vi "ROSmsg_createInd.vi"(9 "Names":string[](array[string]), 11 "SubVI Refnum":refnum<vi>) -> (1 "Exists?":bool, 2 "Control Refnums":refnum<vi>[](array[refnum]), 3 "SubVI Refnum 2":refnum<vi>)   [LabVIEW 2016]
doc: "Creates an indicator for a ROS message"
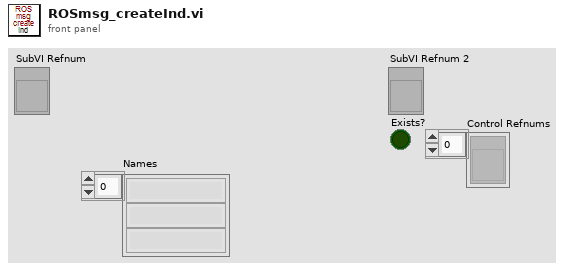
[diagram p1: front panel]
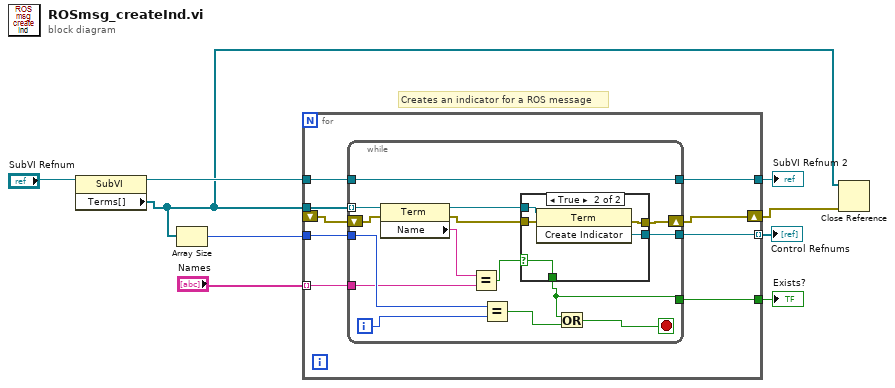
[diagram p0: block diagram]
diagram:
  # "Creates an indicator for a ROS message"
  n1 = property class="SubVI"(reference="SubVI Refnum") -> (reference out=w7:refnum<vi>, "Terms[]"=w1:refnum<vi>[])  [unwired: 1 in, 1 out]
  n2 = Array Size(array=w1) -> (size(s)=w8:i32)
  n3 = for {
    tunnel: w1 -> [w18]
    tunnel: w8 -> [w17]
    tunnel: w7 -> [w16]
    tunnel: [w15] -> w6
    tunnel: [w14] -> w5
    tunnel: [w13] -> w4 mode=indexing
    tunnel: "Names" -> [w12] mode=indexing
    shift-right: [w11] -> w2
    shift-left: _ -> [w10]
    n4 = while {
      tunnel: w18 -> [w33] mode=indexing
      tunnel: w17 -> [w30]
      tunnel: w16 -> [w25]
      tunnel: [w25] -> w15
      tunnel: [w24] -> w13
      tunnel: [w23] -> w14
      tunnel: w12 -> [w22]
      shift-right: [w20] -> w11
      shift-left: w10 -> [w19]
      i -> [w31]
      stop <- w28 stop-if-true
      n5 = property class="Term"(reference=w33, error in=w19) -> (reference out=w26:refnum<vi>, error out=w21:errorcluster, "Name"=w32:string)
      n6 = Equal?(x=w32, y=w22) -> (x = y?=w27:bool)
      n7 = Equal?(x=w30, y=w31) -> (x = y?=w29:bool)
      n8 = case shown="True" w27 {
        selector: w27 -> [w35 w40]
        tunnel: [w35 w40] -> w23
        tunnel: w26 -> [_ w39]
        tunnel: [_ w38] -> w24
        tunnel: w21 -> [w34 w37]
        tunnel: [w34 w36] -> w20
        frame False {
        }
        frame True {
          n9 = invoke class="Term" method="Create Indicator"(reference=w39, error in=w37) -> (error out=w36:errorcluster, "Create Indicator"=w38:refnum<vi>)  [unwired: 1 in, 1 out]
        }
      }
      n10 = Or(x=w23, y=w29) -> (x .or. y?=w28:bool)
    }
  }
  "SubVI Refnum 2" <- w6
  "Exists?" <- w5
  "Control Refnums" <- w4
  n11 = Close Reference(reference=w1, error in (no error)=w2) -> ()  [unwired: 1 out]
